vi "Test_WriteValue_TransportClosed_WriteError.vi"(8 "error in (no error)":errorcluster, 11 "TestCase in":refnum<class "TestQueueTransport.lvclass">) -> (0 "error out":errorcluster, 3 "TestCase out":refnum<class "TestQueueTransport.lvclass">)   [LabVIEW 2017, in "TestQueueTransport.lvclass"]
uses:
  TestQueueTransport.lvclass
  Source/Concrete/QueueTransport/QueueTransport.lvclass
  C:/Git/composed-transport/Source/ITransport/ITransport.lvclass
  Source/ITransport/ITransport.lvclass
panel:
  out "Return Error":errorcluster
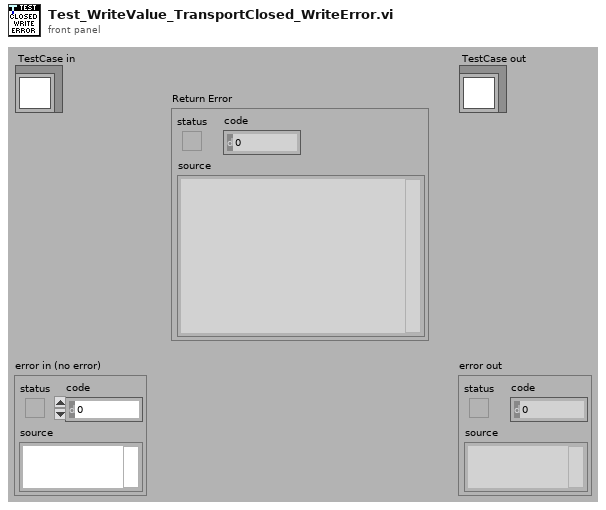
[diagram p1: front panel]
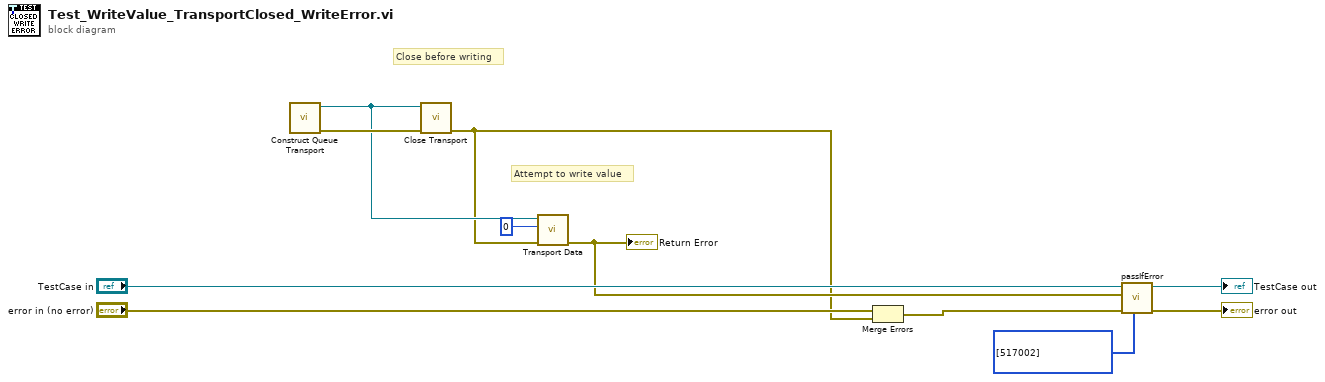
[diagram p0: block diagram]
diagram:
  # "Close before writing"
  # "Attempt to write value"
  n1 = call "Construct Queue Transport.vi"() -> ("error out"=w5:errorcluster, "QueueTransport"=w4:refnum<class "QueueTransport.lvclass">)  [unwired: 10 in]
  n2 = call-dynamic "Close Transport.vi"("error in (no error)"=w5, "QueueTransport"=w4) -> ("error out"=w2:errorcluster)  [unwired: 9 in]
  n3 = call "Transport Data.vi"("error in (no error)"=w2, "Value"=0, "ITransport in"=w4) -> ("error out"=w3:errorcluster)  [unwired: 7 in, 1 out]
  "Return Error" <- w3
  n4 = Merge Errors("error in (no error)", w2) -> (w6:errorcluster)
  n5 = call-dynamic "passIfError.vi"("passing error codes (default = any error code)"=i32[] [517002], "error in (no error)"=w6, "error"=w3, "TestCase in"="TestCase in") -> ("error out"=→"error out":errorcluster, "TestCase out"=→"TestCase out":refnum<class "TestQueueTransport.lvclass">)  [unwired: 6 in]
